vi "R4SBRControl_Status.vi"(7 "LabVIEW Web Service Request":refnum<class "Web Request.lvclass">) -> (0 "error out":errorcluster, 3 "SBRData":T1)   [LabVIEW 2016]
uses:
  <vilib>/wsapi/Web Request.lvclass
  R4Controls/R4SBR_Status.ctl
  R4Controls/R4SBR_SetParams.ctl
panel:
  # "Use the Web Service Request input terminal to call the VIs on the Web Services palette. Do not remove it from the connector pane unless you don't need access to the palette."
  # "Each additional control wired to the connector pane will be available as an input in the URL. To include an indicator in terminal-mode output (the default setting), it must also be wired to the connector pane."
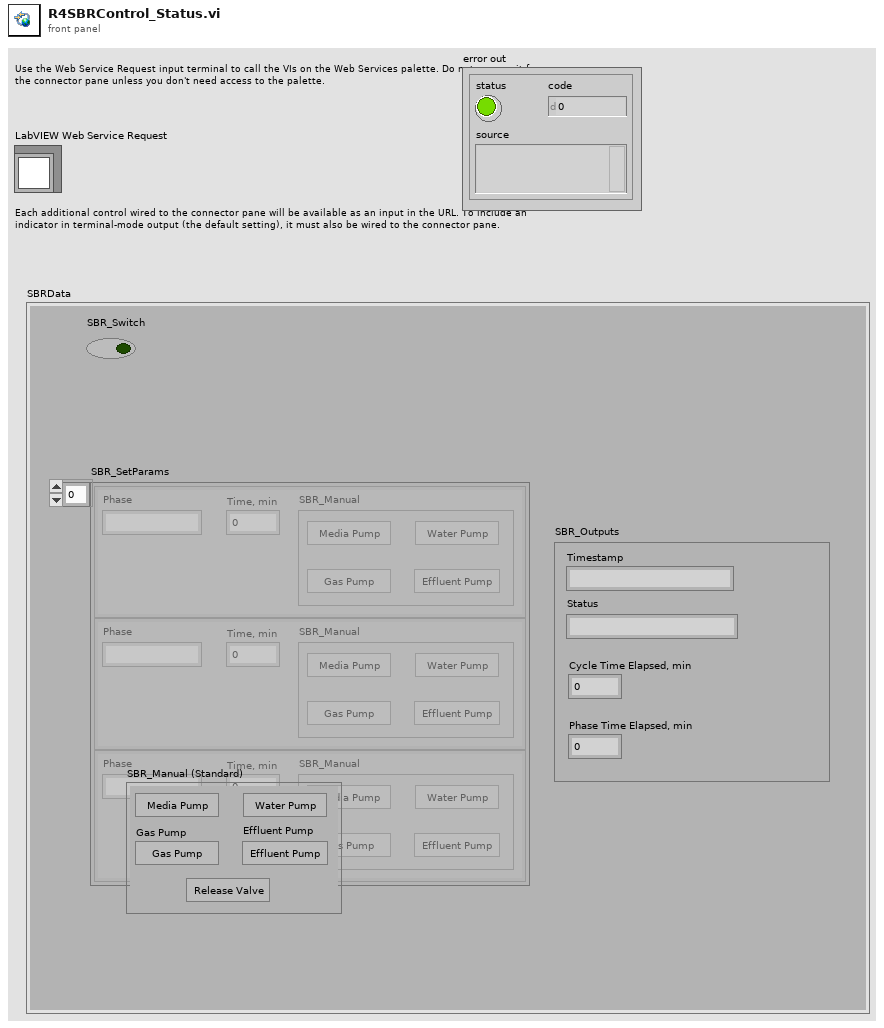
[diagram p1: front panel]
types:
  T1 = typedef "R4SBR_Status.ctl" = cluster{"SBR_Switch":bool, "SBR_Outputs":cluster{"Cycle Time Elapsed, min":dbl, "Phase Time Elapsed, min":dbl, "Timestamp":string, "Status":string}, "SBR_SetParams":T2, "SBR_Manual (Standard)":cluster{"Media Pump":bool, "Water Pump":bool, "Gas Pump":bool, "Effluent Pump":bool, "Release Pump":bool}}
  T2 = typedef "R4SBR_SetParams.ctl" = cluster{"Phase":string, "Time, min":dbl, "SBR_Manual":cluster{"Media Pump":bool, "Water Pump":bool, "Gas Pump":bool, "Effluent Pump":bool}}[]
  T3 = cluster{"Media Pump":bool, "Water Pump":bool, "Gas Pump":bool, "Effluent Pump":bool, "Release Pump":bool}
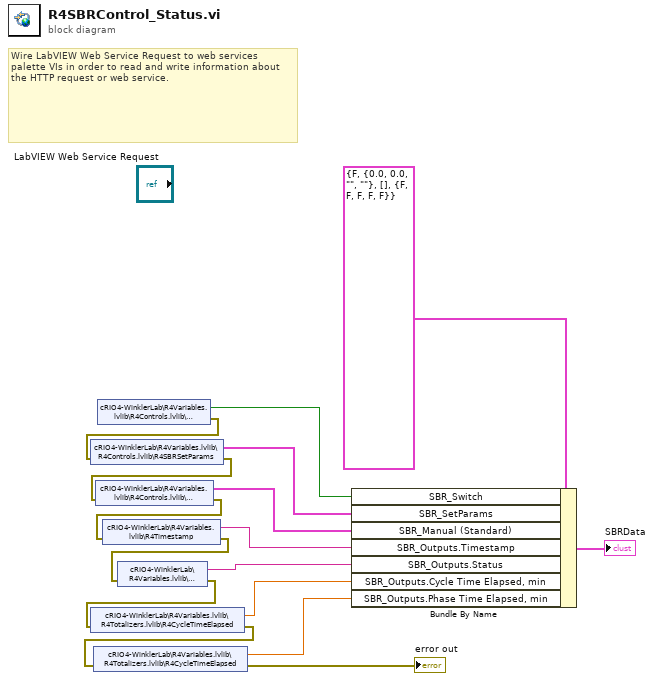
[diagram p0: block diagram]
diagram:
  # "Wire LabVIEW Web Service Request to web services palette VIs in order to read and write information about the HTTP request or web service."
  n1 = shared-variable "cRIO4-WinklerLab\\R4Variables.lvlib\\R4Controls.lvlib\\R4SBRSwitch"() -> (w1:bool, error out=w14:errorcluster)  [unwired: 1 in]
  n2 = shared-variable "cRIO4-WinklerLab\\R4Variables.lvlib\\R4Controls.lvlib\\R4SBRSetParams"(error in=w14) -> (w2:T2, error out=w13:errorcluster)
  n3 = shared-variable "cRIO4-WinklerLab\\R4Variables.lvlib\\R4Controls.lvlib\\R4SBRManual"(error in=w13) -> (w4:T3, error out=w3:errorcluster)
  n4 = shared-variable "cRIO4-WinklerLab\\R4Variables.lvlib\\R4Timestamp"(error in=w3) -> (w5:string, error out=w12:errorcluster)
  n5 = shared-variable "cRIO4-WinklerLab\\R4Variables.lvlib\\R4Status"(error in=w12) -> (w6:string, error out=w11:errorcluster)
  n6 = shared-variable "cRIO4-WinklerLab\\R4Variables.lvlib\\R4Totalizers.lvlib\\R4CycleTimeElapsed"(error in=w11) -> (w7:dbl, error out=w10:errorcluster)
  n7 = shared-variable "cRIO4-WinklerLab\\R4Variables.lvlib\\R4Totalizers.lvlib\\R4CycleTimeElapsed"(error in=w10) -> (w9:dbl, error out=→"error out":errorcluster)
  n8 = Bundle By Name(cluster=T1 {"SBR_Switch"=FALSE, "SBR_Outputs"={"Cycle Time Elapsed, min"=0.0, "Phase Time Elapsed, min"=0.0, "Timestamp"="", "Status"=""}, "SBR_SetParams"=[], "SBR_Manual (Standard)"={"Media Pump"=FALSE, "Water Pump"=FALSE, "Gas Pump"=FALSE, "Effluent Pump"=FALSE, "Release Pump"=FALSE}} ("SBRData"), "SBR_Switch"=w1, "SBR_SetParams"=w2, "SBR_Manual (Standard)"=w4, "SBR_Outputs.Timestamp"=w5, "SBR_Outputs.Status"=w6, "SBR_Outputs.Cycle Time Elapsed, min"=w7, "SBR_Outputs.Phase Time Elapsed, min"=w9) -> (→"SBRData":T1)
